vi "RTEH Get Next Error.vi"() -> (0 "Internal Error":errorcluster, 1 "Transmitted Error":errorcluster, 2 "Empty?":bool, 3 "Notification Info":T1, 5 "Classification":u32)   [LabVIEW 2017]
doc: "Returns an error notification from the nofication queue. Notifications are enqueued using the Specific Error Handler.\n\nThis VI is optimized for Real-Time applications. An alternate version for Windows VIs exists."
uses:
  <userlib>/_SEH/Controls/Shared/SEH Notification Info.ctl
  <userlib>/_SEH/Controls/Shared/SEH Error Notification Command.ctl
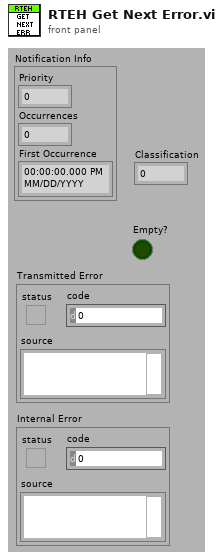
[diagram p1: front panel]
types:
  T1 = typedef "SEH Notification Info.ctl" = cluster{"Priority":i32, "Occurrences":i32, "First Occurrence":timestamp}
  T2 = typedef "SEH Error Notification Command.ctl" = enum16{"Init", "Send Error", "Check Error", "Invalid Command"}
  T3 = typedef "RTEH Status Type.ctl" = enum16{"Success", "Error", "Warning", "Skipped Notification"}
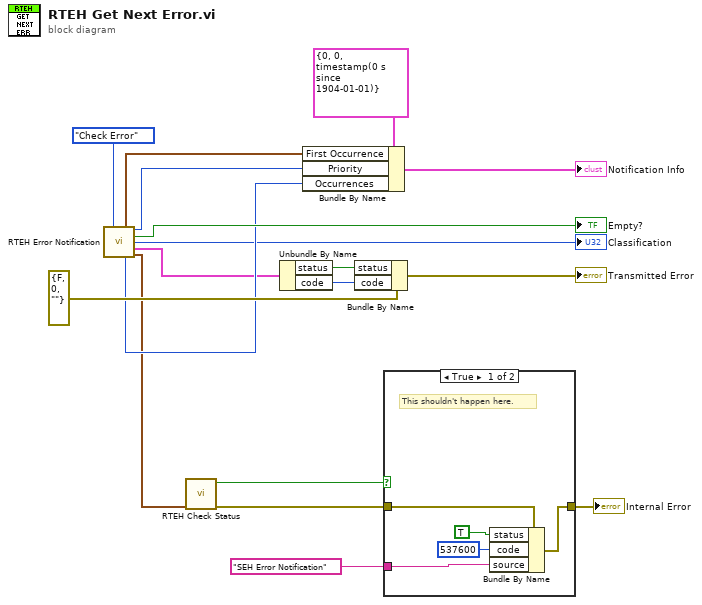
[diagram p0: block diagram]
diagram:
  n1 = call <userlib>:"RTEH Error Notification.vi"("Command"=SEH_Error_Notification_Command."Check Error") -> ("First Occurrence"=w12:timestamp, "Priority Out"=w11:i32, "Empty?"=→"Empty?":bool, "Classification Out"=→"Classification":u32, "Transmitted Error"=w6:cluster{"status":bool, "code":i32}, "Occurrences"=w10:i32, "Internal Status"=w5:cluster{"Status":T3, "Error Code":i32})  [unwired: 7 in, 1 out]
  n2 = call <userlib>:"RTEH Check Status.vi"("Internal Status"=w5) -> ("Internal Error"=w1:errorcluster, "Skipped"=w4:bool)  [unwired: 9 in]
  n3 = Unbundle By Name(w6) -> ("status"=w14:bool, "code"=w13:i32)
  n4 = Bundle By Name(cluster=T1 {"Priority"=0, "Occurrences"=0, "First Occurrence"=timestamp(0 s since 1904-01-01)} ("Notification Info"), "First Occurrence"=w12, "Priority"=w11, "Occurrences"=w10) -> (→"Notification Info":T1)
  n5 = Bundle By Name(cluster=errorcluster {"status"=FALSE, "code"=0, "source"=""} ("Transmitted Error"), "status"=w14, "code"=w13) -> (→"Transmitted Error":errorcluster)
  n6 = case shown="True" w4 {
    tunnel: w1 -> [w23 w24]
    tunnel: "SEH Error Notification" ("source") -> [w21 _]
    tunnel: [w22 w24] -> w2
    frame True {
      # "This shouldn't happen here."
      n7 = Bundle By Name(cluster=w23, "status"=TRUE, "code"=537600, "source"=w21) -> (w22:errorcluster)
    }
    frame False {
    }
  }
  "Internal Error" <- w2
